vi "test_FPGAWrapperAN110607Galvo.vi"() -> ()   [LabVIEW 2010, in "FPGAWrapperAN110607Galvo.lvclass"]
uses:
  FPGAWrapperAN110607Galvo.lvclass
  common/classes/ErrorController/ErrorController/ErrorController.lvclass
  common/classes/ErrorController/ErrorController/class_data.vi
panel:
  in  "gate parameters":T1
  in  "number of channels":i32=2
  in  "milliseconds to wait":u32(slide) scale=0.0..200.0
  out "samples read":i64
  in  "pixel frequency":dbl[unit]=250000.0
  out "pixel dwell time":dbl[unit]
  in  "number of pixels":i32=1000000000
  in  "run button":bool
  in  "create button":bool
  in  "stop":bool
  out "AN110607FPGAWrapper out":refnum<class "FPGAWrapperAN110607Galvo.lvclass">
  in  "block size":i32=16000
  out "channel data block":dbl[][](graph)
  in  "timeout (ms)":i32=500
  out "timed out?":bool
  out "DAQ loop counter":i32
  out "error controller loaded?":bool=TRUE
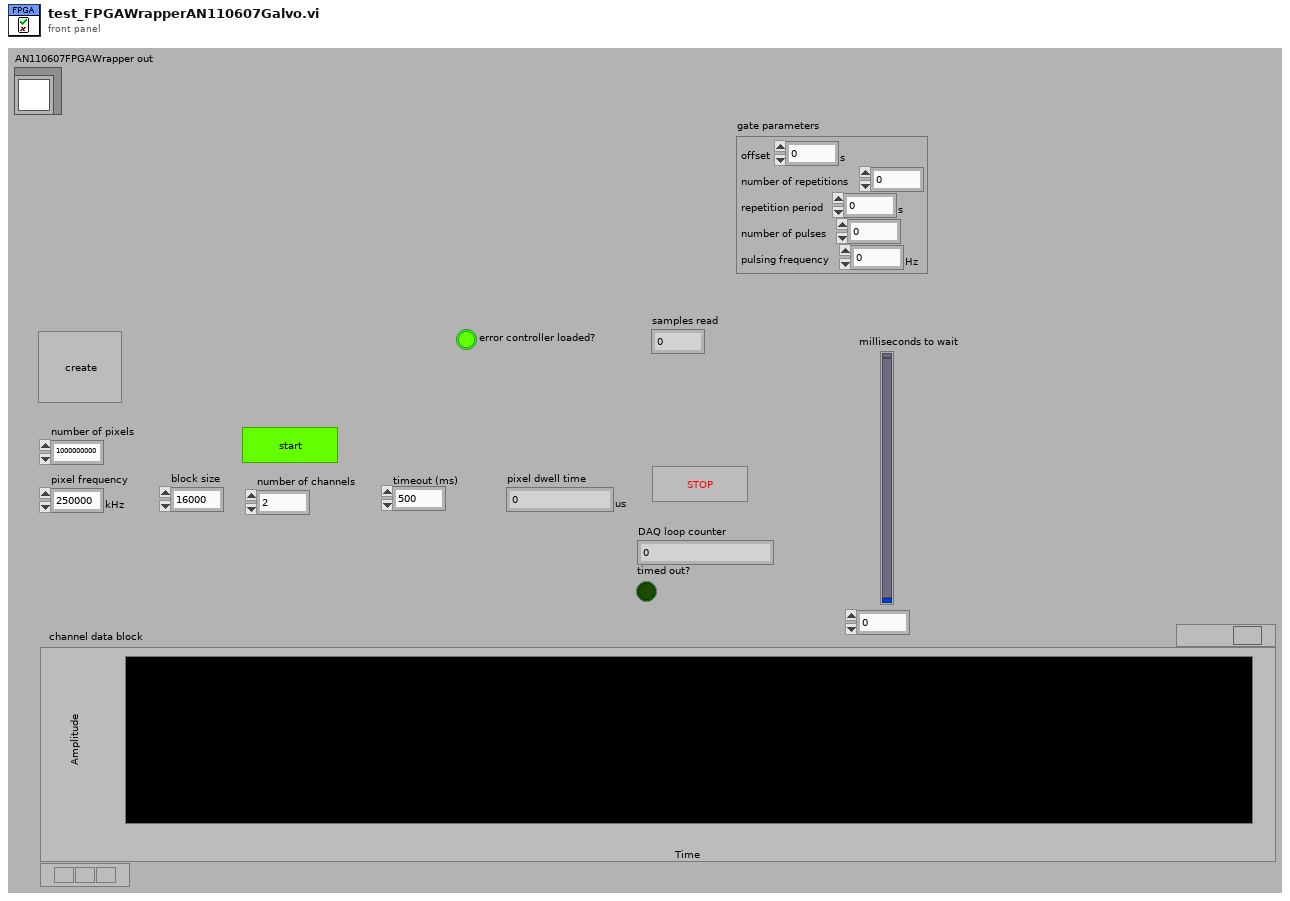
[diagram p1: front panel]
types:
  T1 = cluster{"offset":dbl[unit], "number of repetitions":i64, "repetition period":dbl[unit], "number of pulses":i64, "pulsing frequency":dbl[unit]}
  T2 = typedef "plugin_specification.ctl" = cluster{"class path":string, "configuration":string, "label":string, "settings name":string}
  T3 = typedef "XComponentSpecification.xctl/data.ctl" = cluster{"class path":string, "configuration":string, "label":string, "settings name":string}
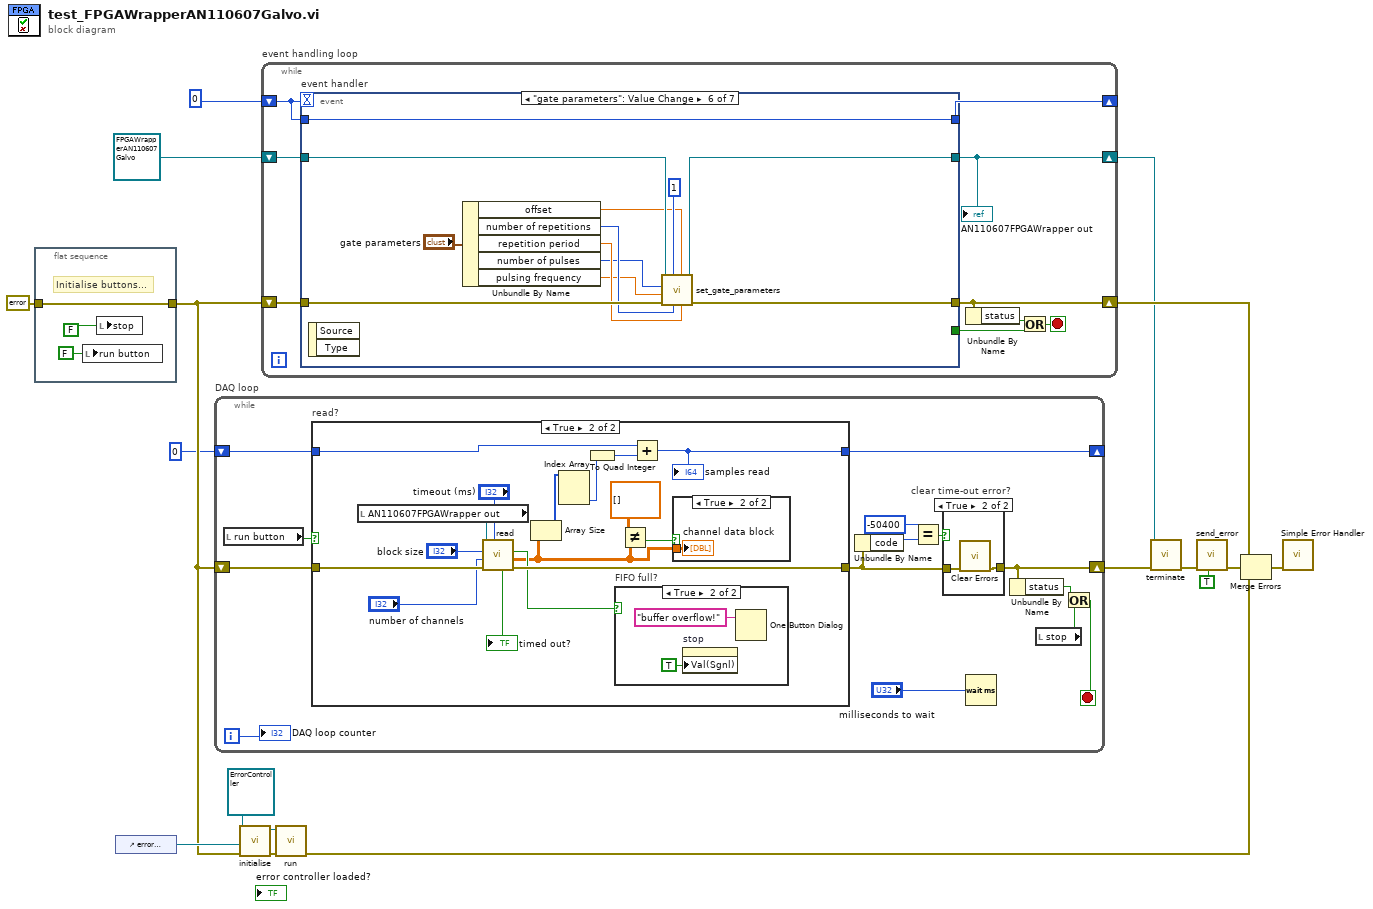
[diagram p0: block diagram]
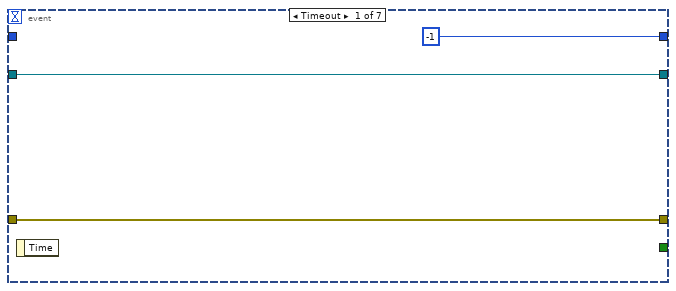
[diagram p6: hidden frame]
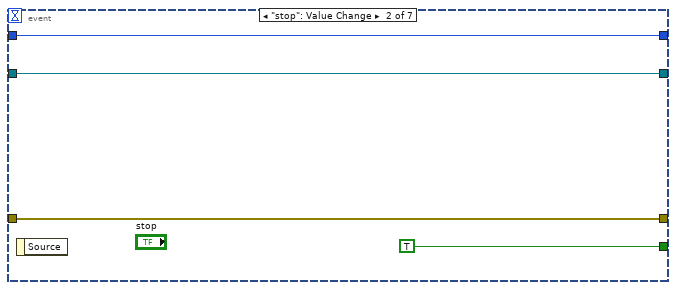
[diagram p7: hidden frame]
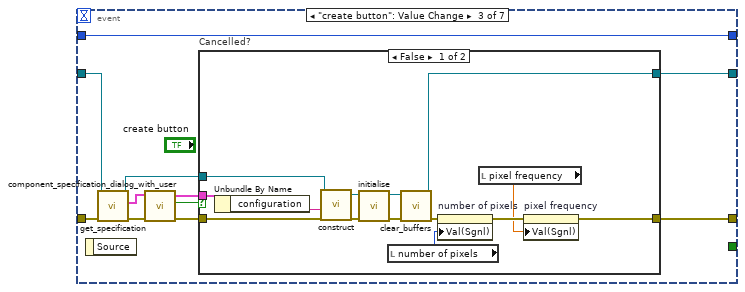
[diagram p8: hidden frame]
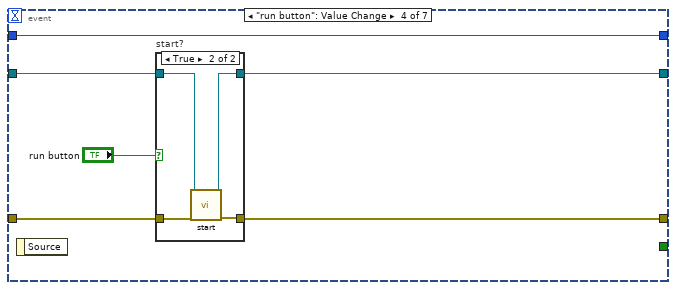
[diagram p10: hidden frame]
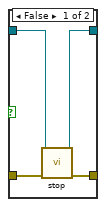
[diagram p11: hidden frame]
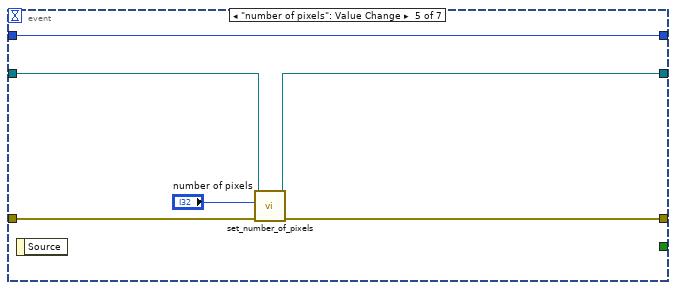
[diagram p12: hidden frame]
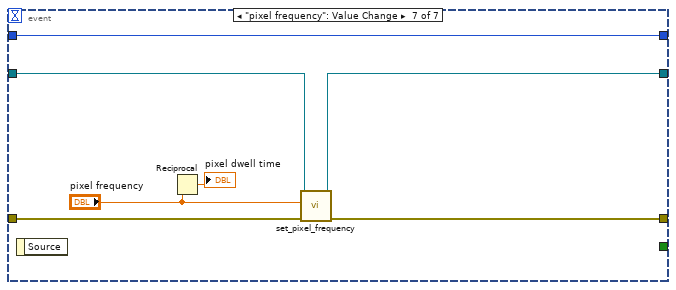
[diagram p13: hidden frame]
diagram:
  n1 = flat-sequence {
    tunnel: errorcluster {"status"=FALSE, "code"=0, "source"=""} ("error in (no error)") -> [w20]
    tunnel: [w20] -> w12
    frame #0 {
      # "Initialise buttons..."
      n2 = local write "run button"(FALSE ("run button")) -> ()
      n3 = local write "stop"(FALSE) -> ()
    }
  }
  n4 = control-ref of="error controller loaded?"() -> (w17:refnum<vi>)
  n5 = while "DAQ loop" {
    shift-right: [w28] -> w5
    shift-left: w12 -> [w34]
    shift-right: [w22] -> _
    shift-left: i64 0 -> [w23]
    i -> [w24]
    stop <- w25 stop-if-true
    n6 = local read "run button"() -> (w33:bool)
    n7 = case "read?" shown="True" w33 {
      tunnel: w34 -> [w38 w54]
      tunnel: [w38 w53] -> w30
      tunnel: w23 -> [_ w45]
      tunnel: [_ w44] -> w22
      frame False {
      }
      frame True {
        n8 = local read "AN110607FPGAWrapper out"() -> (w52:refnum<class "FPGAWrapperAN110607Galvo.lvclass">)
        n9 = call-dynamic "read.vi"("timeout (ms)"="timeout (ms)", "error in (no error)"=w54, "number of channels"="number of channels", "block size"="block size", "FPGAWrapperAN110607Galvo in"=w52) -> ("error out"=w53:errorcluster, "data"=w46:dbl[][], "FIFO full?"=w48:bool, "timed out?"=→"timed out?":bool)  [unwired: 3 out]
        n10 = Array Size(array=w46) -> (size(s)=w42:i32[])
        n11 = Index Array(array=w42) -> (element #2=w41:i32)  [unwired: 2 in, 1 out]
        n12 = To Quad Integer(1:w41) -> (0:w40:i64)
        n13 = case "FIFO full?" shown="True" w48 {
          frame False {
          }
          frame True {
            n14 = property on="stop" class="Bool (strict)"("Val(Sgnl)"=TRUE) -> ()  [unwired: 2 in, 2 out]
            n15 = One Button Dialog(message="buffer overflow!") -> ()  [unwired: 1 in, 1 out]
          }
        }
        n16 = Not Equal?(x=dbl[][] [], y=w46) -> (x != y?=w50:bool)
        n17 = Add(x=w45, y=w40) -> (x+y=w44:i64)
        "samples read" <- w44
        n18 = case shown="True" w50 {
          tunnel: w46 -> [_ w57]
          frame False {
          }
          frame True {
            "channel data block" <- w57
          }
        }
      }
    }
    n19 = Unbundle By Name(w30) -> ("code"=w32:i32)
    n20 = Equal?(x=-50400, y=w32) -> (x = y?=w29:bool)
    n21 = case "clear time-out error?" shown="True" w29 {
      tunnel: w30 -> [w35 w37]
      tunnel: [w35 w36] -> w28
      frame False {
      }
      frame True {
        n22 = call <vilib>:"Clear Errors.vi"("error in (no error)"=w37) -> ("error out"=w36:errorcluster)  [unwired: 6 out]
      }
    }
    n23 = Wait (ms)(milliseconds to wait="milliseconds to wait") -> ()  [unwired: 1 out]
    n24 = Unbundle By Name(w28) -> ("status"=w27:bool)
    n25 = local read "stop"() -> (w26:bool)
    n26 = Or(x=w27, y=w26) -> (x .or. y?=w25:bool)
    "DAQ loop counter" <- w24
  }
  n27 = call-dynamic "initialise.vi"("error in (no error)"=w12, "error boolean"=w17, "ErrorController in"=refnum<class "ErrorController.lvclass"> refnum) -> ("error out"=w9:errorcluster, "ErrorController out"=w10:refnum<class "ErrorController.lvclass">)  [unwired: 7 in]
  n28 = while "event handling loop" {
    shift-right: [w61] -> w7
    shift-left: w12 -> [w66]
    shift-right: [w64] -> _
    shift-left: 0 -> [w65]
    shift-right: [w62] -> w6
    shift-left: refnum<class "FPGAWrapperAN110607Galvo.lvclass"> refnum ("FPGAWrapperAN110607Galvo.lvclass") -> [w63]
    stop <- w58 stop-if-true
    n29 = event "event handler" shown="[5] \"gate parameters\": Value Change" {
      selector: _ -> [_ _ _ _ _ _ _]
      dyn-events: _ -> [_ _ _ _ _ _ _]
      timeout: w65 -> [_ _ _ _ _ _ _]
      tunnel: [w67 w70 w83 w102 w118 w130 w137] -> w61
      tunnel: w66 -> [w67 w70 w80 w105 w119 w131 w138]
      tunnel: w65 -> [_ w73 w84 w106 w120 w132 w139]
      tunnel: [-1 w73 w84 w106 w120 w132 w139] -> w64
      tunnel: [_ TRUE _ _ _ _ _] -> w59
      tunnel: [w68 w71 w75 w103 w116 w128 w135] -> w62
      tunnel: w63 -> [w68 w71 w78 w104 w117 w129 w136]
      event Timeout {
        n30 = event-data() -> ()  [unwired: 2 out]
      }
      event "stop": Value Change {
        n31 = event-data() -> ()  [unwired: 2 out]
      }
      event "create button": Value Change {
        n32 = event-data() -> ()  [unwired: 2 out]
        n33 = call-dynamic "get_specification.vi"("error in (no error)"=w80, "GenericPlugin in"=w78) -> ("error out"=w79:errorcluster, "component specification"=w76:T2, "GenericPlugin out"=w77:refnum<class "FPGAWrapperAN110607Galvo.lvclass">)  [unwired: 6 in, 1 out]
        n34 = call "component_specification_dialog_with_user.vi"("error in (no error)"=w79, "component specification in"=w76) -> ("error out"=w82:errorcluster, "cancelled?"=w74:bool, "component specification out"=w81:T3)  [unwired: 7 in]
        n35 = case "Cancelled?" shown="False" w74 {
          tunnel: [w85 w100] -> w83
          tunnel: w82 -> [w90 w100]
          tunnel: w81 -> [w89 _]
          tunnel: w77 -> [w87 w99]
          tunnel: [w86 w99] -> w75
          frame False {
            n36 = Unbundle By Name(w89) -> ("configuration"=w88:string)
            n37 = call-dynamic "construct.vi"("error in (no error)"=w90, "configuration name"=w88, "GenericPlugin in"=w87) -> ("error out"=w92:errorcluster, "GenericPlugin out"=w91:refnum<class "FPGAWrapperAN110607Galvo.lvclass">)  [unwired: 7 in]
            n38 = call-dynamic "initialise.vi"("error in (no error)"=w92, "GenericPlugin in"=w91) -> ("error out"=w95:errorcluster, "GenericPlugin out"=w93:refnum<class "FPGAWrapperAN110607Galvo.lvclass">)  [unwired: 1 in, 7 out]
            n39 = local read "number of pixels"() -> (w96:i32)
            n40 = call-dynamic "clear_buffers.vi"("error in (no error)"=w95, "FPGAWrapperAN110607Galvo in"=w93) -> ("error out"=w94:errorcluster, "FPGAWrapperAN110607Galvo out"=w86:refnum<class "FPGAWrapperAN110607Galvo.lvclass">)  [unwired: 8 in]
            n41 = property on="number of pixels" class="DigNum (strict)"(error in=w94, "Val(Sgnl)"=w96) -> (error out=w98:errorcluster)  [unwired: 1 in, 1 out]
            n42 = local read "pixel frequency"() -> (w97:dbl[unit])
            n43 = property on="pixel frequency" class="DigNum (strict)"(error in=w98, "Val(Sgnl)"=w97) -> (error out=w85:errorcluster)  [unwired: 1 in, 1 out]
          }
          frame True {
          }
        }
      }
      event "run button": Value Change {
        n44 = event-data() -> ()  [unwired: 2 out]
        n45 = case "start?" shown="True" "run button" {
          tunnel: w105 -> [w110 w114]
          tunnel: w104 -> [w108 w113]
          tunnel: [w107 w112] -> w103
          tunnel: [w109 w111] -> w102
          frame False {
            n46 = call-dynamic "stop.vi"("error in (no error)"=w110, "FPGAWrapperAN110607Galvo in"=w108) -> ("error out"=w109:errorcluster, "FPGAWrapperAN110607Galvo out"=w107:refnum<class "FPGAWrapperAN110607Galvo.lvclass">)  [unwired: 8 out]
          }
          frame True {
            n47 = call-dynamic "start.vi"("error in (no error)"=w114, "FPGAWrapperAN110607Galvo in"=w113) -> ("error out"=w111:errorcluster, "FPGAWrapperAN110607Galvo out"=w112:refnum<class "FPGAWrapperAN110607Galvo.lvclass">)  [unwired: 8 out]
          }
        }
      }
      event "number of pixels": Value Change {
        n48 = event-data() -> ()  [unwired: 2 out]
        n49 = call-dynamic "set_number_of_pixels.vi"("error in (no error)"=w119, "number of pixels"="number of pixels", "FPGAWrapperAN110607Galvo in"=w117) -> ("error out"=w118:errorcluster, "FPGAWrapperAN110607Galvo out"=w116:refnum<class "FPGAWrapperAN110607Galvo.lvclass">)  [unwired: 7 out]
      }
      event "gate parameters": Value Change {
        n50 = event-data() -> ()  [unwired: 3 out]
        n51 = Unbundle By Name("gate parameters") -> ("offset"=w125:dbl[unit], "number of repetitions"=w124:i64, "repetition period"=w123:dbl[unit], "number of pulses"=w122:i64, "pulsing frequency"=w121:dbl[unit])
        n52 = call-dynamic "set_gate_parameters.vi"("repetition period"=w123, "offset"=w125, "number of repetitions"=w124, "clock index"=1, "error in (no error)"=w131, "pulsing frequency"=w121, "number of pulses"=w122, "FPGAWrapperAN110607Galvo in"=w129) -> ("error out"=w130:errorcluster, "FPGAWrapperAN110607Galvo out"=w128:refnum<class "FPGAWrapperAN110607Galvo.lvclass">)  [unwired: 2 in]
      }
      event "pixel frequency": Value Change {
        n53 = event-data() -> ()  [unwired: 2 out]
        n54 = Reciprocal(x="pixel frequency") -> (1/x=→"pixel dwell time":dbl[unit])
        n55 = call-dynamic "set_pixel_frequency.vi"("error in (no error)"=w138, "pixel frequency"="pixel frequency", "FPGAWrapperAN110607Galvo in"=w136) -> ("error out"=w137:errorcluster, "FPGAWrapperAN110607Galvo out"=w135:refnum<class "FPGAWrapperAN110607Galvo.lvclass">)  [unwired: 7 in]
      }
    }
    "AN110607FPGAWrapper out" <- w62
    n56 = Unbundle By Name(w61) -> ("status"=w60:bool)
    n57 = Or(x=w60, y=w59) -> (x .or. y?=w58:bool)
  }
  n58 = call "run.vi"("error in (no error)"=w9, "ErrorController in"=w10) -> ("error out"=w16:errorcluster)  [unwired: 8 in, 1 out]
  n59 = call-dynamic "terminate.vi"("error in (no error)"=w5, "GenericPlugin in"=w6) -> ("error out"=w13:errorcluster)  [unwired: 9 out]
  n60 = call "send_error.vi"("last error? (F)"=TRUE, "error in (no error)"=w13) -> ("error out"=w14:errorcluster)  [unwired: 9 in]
  n61 = Merge Errors(w7, w14, w16) -> (w8:errorcluster)
  n62 = call <vilib>:"Simple Error Handler.vi"("error in (no error)"=w8) -> ()  [unwired: 1 in, 8 out]
